vi "BGA244_meas_ratio.vi"(8 "error in":errorcluster, 11 "VISA in":refnum<visa-resource-name>) -> (0 "error out":errorcluster, 1 "ratio2":dbl, 2 "ratio1":dbl, 3 "VISA out":refnum<visa-resource-name>, 4 "status":bool)   [LabVIEW 2019]
panel:
  out "string 2":string
  out "string 1":string
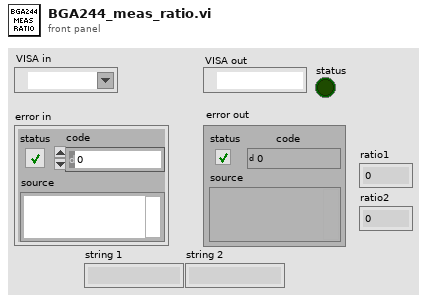
[diagram p1: front panel]
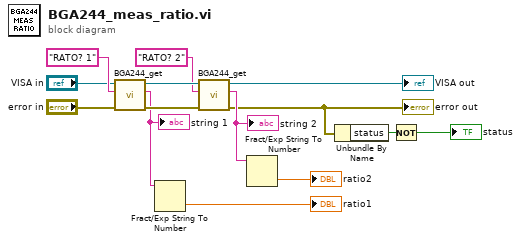
[diagram p0: block diagram]
diagram:
  n1 = call "BGA244_get.vi"("error in"="error in", "string in"="RATO? 1" ("string"), "VISA in"="VISA in") -> ("error out"=w9:errorcluster, "string out"=w6:string, "VISA out"=w11:refnum<visa-resource-name>)  [unwired: 6 in]
  "string 1" <- w6
  n2 = Fract/Exp String To Number(string=w6) -> (number=→"ratio1":dbl)  [unwired: 3 in, 1 out]
  n3 = call "BGA244_get.vi"("error in"=w9, "string in"="RATO? 2" ("string"), "VISA in"=w11) -> ("error out"=w4:errorcluster, "string out"=w7:string, "VISA out"=→"VISA out":refnum<visa-resource-name>)  [unwired: 6 in]
  "error out" <- w4
  "string 2" <- w7
  n4 = Fract/Exp String To Number(string=w7) -> (number=→"ratio2":dbl)  [unwired: 3 in, 1 out]
  n5 = Unbundle By Name(w4) -> ("status"=w5:bool)
  n6 = Not(x=w5) -> (.not. x?=→"status":bool)
